vi "Get Active UI Function.vi"(0 "UI Functions in":refnum<class "UI Functions.lvclass">, 11 "error in (no error)":errorcluster) -> (4 "UI Functions out":refnum<class "UI Functions.lvclass">, 6 "Function List":T1, 15 "error out":errorcluster)   [LabVIEW 2019, in "UI Functions.lvclass"]
uses:
  UI Functions.lvclass
  D:/Pet Projects/LSL/source code/LSL components/functions/functionsbase/functionbase.lvclass
  Function List.ctl
  functionsbase/functionbase.lvclass
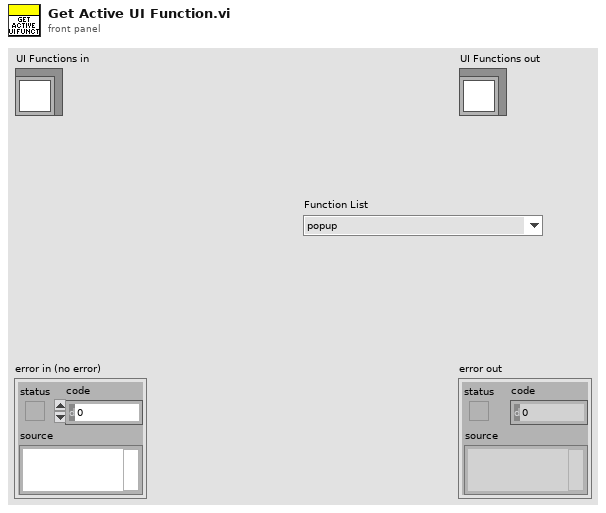
[diagram p1: front panel]
types:
  T1 = typedef "UI Functions.lvclass/Function List.ctl" = enum16{"popup", "print", "Get Bool", "Get Number", "Get String"}
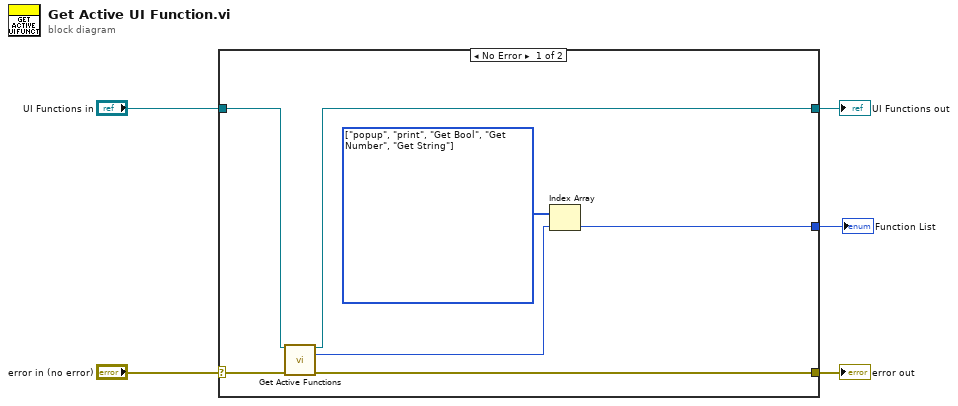
[diagram p0: block diagram]
diagram:
  n1 = case shown="No Error" "error in (no error)" {
    selector: "error in (no error)" -> [w12 w14]
    tunnel: [w11 w14] -> w4
    tunnel: [w9 w13] -> w2
    tunnel: "UI Functions in" -> [w10 w13]
    tunnel: [w6 _] -> w1
    frame No Error {
      w8 = T1[] [enum."popup", enum."print", enum."Get Bool", enum."Get Number", enum."Get String"] items=["popup", "print", "Get Bool", "Get Number", "Get String"]
      n2 = call "Get Active Functions.vi"("functionbase in"=w10, "error in (no error)"=w12) -> ("functionbase out"=w9:refnum<class "UI Functions.lvclass">, "Syntax Index"=w7:i32, "error out"=w11:errorcluster)  [unwired: 11 in]
      n3 = Index Array(array=w8, index=w7) -> (element=w6:T1)
    }
    frame Error {
    }
  }
  "error out" <- w4
  "UI Functions out" <- w2
  "Function List" <- w1
